vi "ParserCode.vi"(11 "ArgumentParser in":refnum<class "ArgumentParser.lvclass">) -> (2 "ParserCode":string, 3 "ArgumentParser out":refnum<class "ArgumentParser.lvclass">)   [LabVIEW 2022 SP3, in "ArgumentParser.lvlib" / "ArgumentParser.lvclass"]
uses:
  ArgumentParser.lvclass
  ArgumentParser.lvclass/ArgumentParser.ctl
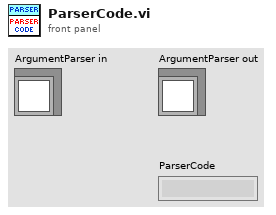
[diagram p1: front panel]
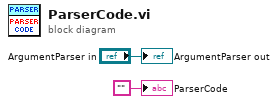
[diagram p0: block diagram]
diagram:
  "ArgumentParser out" <- "ArgumentParser in"
  "ParserCode" <- ""
